vi "Example Callback.vi"() -> ()   [LabVIEW 2010]
uses:
  C:/tf/play/labview/Tinkerforge.dll
  Tinkerforge.dll
panel:
  in  "stop":bool
  out "voltage (V)":sgl format="%#_13g"
  in  "uid":string="amb"
  in  "port":i32=4223
  in  "host":string="localhost"
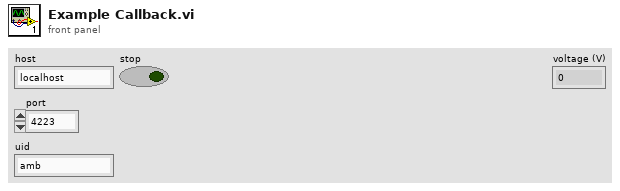
[diagram p1: front panel]
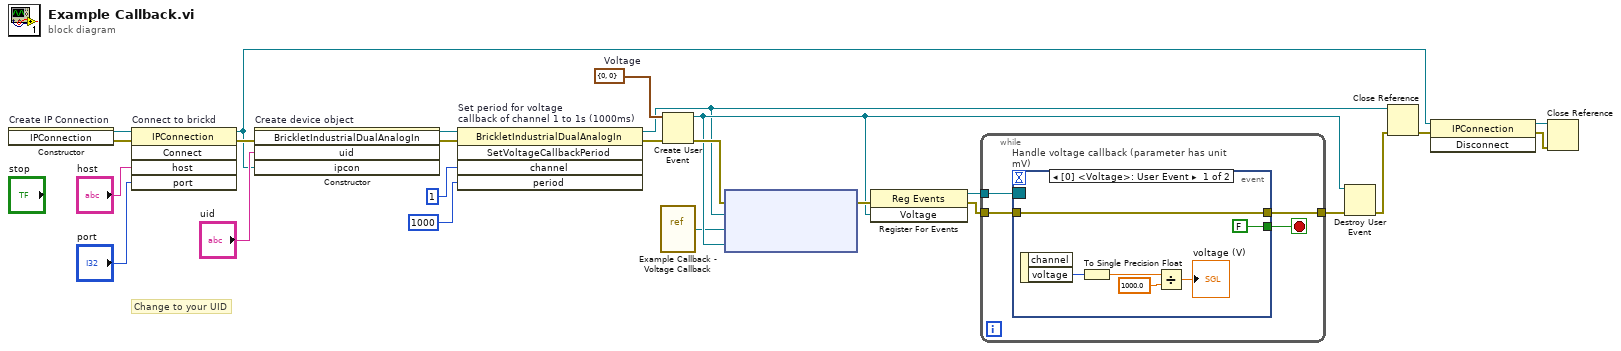
[diagram p0: block diagram]
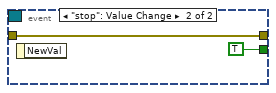
[diagram p2: hidden frame]
diagram:
  w9 = cluster{"channel":u8, "voltage":i32} {"channel"=0, "voltage"=0}  # Voltage
  # "Change to your UID"
  n1 = constructor on="Create IP Connection" class="IPConnection"() -> (reference out=w25:refnum<k24>, error out=w4:errorcluster)  [unwired: 3 in, 1 out]
  n2 = invoke on="Connect to brickd" class="IPConnection" method="Connect"(reference=w25, error in=w4, "host"="host", "port"="port") -> (reference out=w18:refnum<k24>, error out=w21:errorcluster)  [unwired: 1 in, 3 out]
  n3 = constructor on="Create device object" class="BrickletIndustrialDualAnalogIn"(error in=w21, "uid"="uid", "ipcon"=w18) -> (reference out=w6:refnum<k24>, error out=w8:errorcluster)  [unwired: 2 in, 3 out]
  n4 = invoke on="Set period for voltage\ncallback of channel 1 to 1s (1000ms)" class="BrickletIndustrialDualAnalogIn" method="SetVoltageCallbackPeriod"(reference=w6, error in=w8, "channel"=u8 1 ("sensor"), "period"=i64 1000) -> (reference out=w5:refnum<k24>, error out=w7:errorcluster)  [unwired: 1 in, 3 out]
  n5 = vi-ref "Example Callback - Voltage Callback.vi"() -> ("vi reference"=w1:refnum<vi>)
  n6 = Create User Event(user event datatype=w9, error in=w7) -> (user event=w11:refnum<user-event>, error out=w16:errorcluster)
  n7 = node ("Register Event Callback")(w16, w5, w1, w11) -> (w15:errorcluster)  [unwired: 1 in, 1 out]
  n8 = register-events(error in=w15, w11) -> (reference out=w14:refnum<event-registration>, error out=w12:errorcluster)  [unwired: 1 in]
  n9 = while {
    tunnel: w14 -> [w29]
    tunnel: [w28] -> w13
    tunnel: w12 -> [w27]
    stop <- w26 stop-if-true
    n10 = event "Handle voltage callback (parameter has unit mV)" shown="[0] <Voltage>: User Event" {
      selector: w29 -> [_ _]
      dyn-events: _ -> [_ _]
      timeout: _ -> [_ _]
      tunnel: [w32 w36] -> w28
      tunnel: w27 -> [w32 w36]
      tunnel: [FALSE TRUE] -> w26
      event User Event {
        n11 = event-data() -> ("voltage"=w33:i32)  [unwired: 1 in, 1 out]
        n12 = To Single Precision Float(number=w33) -> (single precision float=w34:sgl)
        n13 = Divide(x=w34, y=sgl 1000.0) -> (x/y=→"voltage (V)":sgl)
      }
      event "stop": Value Change {
        n14 = event-data() -> ()  [unwired: 1 in, 1 out]
      }
    }
  }
  n15 = Destroy User Event(user event=w11, error in=w13) -> (error out=w10:errorcluster)
  n16 = Close Reference(reference=w5, error in (no error)=w10) -> (error out=w20:errorcluster)
  n17 = invoke class="IPConnection" method="Disconnect"(reference=w18, error in=w20) -> (reference out=w17:refnum<k24>, error out=w19:errorcluster)  [unwired: 1 in, 1 out]
  n18 = Close Reference(reference=w17, error in (no error)=w19) -> ()  [unwired: 1 out]
